vi "testUnflattenAccelerationFromXML.vi"() -> ()   [LabVIEW 2012, in "UnitsAndXML.lvlib"]
uses:
  <userlib>/Common/UnitsAndXML/UnitsAndXML.lvlib
  <userlib>/Common/UnitsAndXML/FlattenItemWithUnitToXML/FlattenAccelerationToXML/AccelerationUnit.ctl
  <userlib>/Common/UnitsAndXML/UnflattenItemWithUnitFromXML/UnflattenAccelerationFromXML/typeMethods/unflattenAccelerationFromXML_Array.vi
  <userlib>/Common/UnitsAndXML/UnflattenItemWithUnitFromXML/UnflattenAccelerationFromXML/typeMethods/unflattenAccelerationFromXML_Scalar.vi
panel:
  out "error out":errorcluster
  out "acceleration":dbl[unit][](array[numeric])
  out "acceleration":dbl[unit]
  in  "accelerationUnitInXML":T1
  in  "xmlStringArray":string="<acceleration>15</acceleration>\r\n<acceleration>30</acceleration>\r\n<acceleration>45</acceleration>\r\n<acceleration>60</acceleration>"
  in  "xmlStringScalar":string="<acceleration>15</acceleration>"
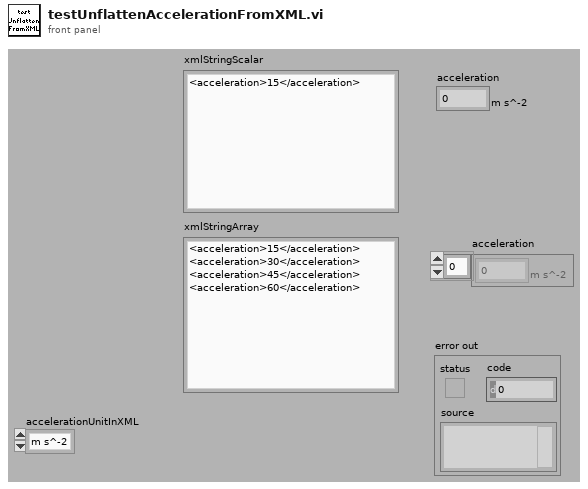
[diagram p1: front panel]
types:
  T1 = typedef "UnitsAndXML.lvlib/AccelerationUnit.ctl" = enum16{"m s^-2"}
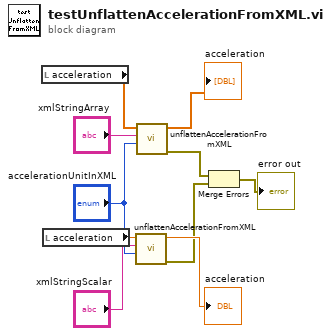
[diagram p0: block diagram]
diagram:
  n1 = local read "acceleration"() -> (w3:dbl[unit][])
  n2 = local read "acceleration"() -> (w9:dbl[unit])
  n3 = call-poly <userlib>:"unflattenAccelerationFromXML.vi"("accelerationUnitInXML"="accelerationUnitInXML", "xmlString"="xmlStringScalar", "accelerationForType"=w9) -> ("error out"=w5:errorcluster, "acceleration"=→"acceleration":dbl[unit])  [unwired: 7 in]
  n4 = call-poly <userlib>:"unflattenAccelerationFromXML.vi"("accelerationUnitInXML"="accelerationUnitInXML", "xmlString"="xmlStringArray", "accelerationForType"=w3) -> ("error out"=w6:errorcluster, "acceleration"=→"acceleration":dbl[unit][])  [unwired: 7 in]
  n5 = Merge Errors(w6, w5) -> (→"error out":errorcluster)
